vi "LDRLouise.vi"() -> ()   [LabVIEW 2015]
uses:
  <vilib>/Math Plots/2D Math Plots/2D Compass/2D Compass XCtrl/2D Compass.xctl
  <vilib>/Math Plots/2D Math Plots/2D Compass/2D Compass Datatype/Public/Plot Helper (Complex).vi
  <vilib>/Math Plots/2D Math Plots/2D Compass/2D Compass Datatype/2D Compass Datatype.lvclass
panel:
  out "2D Compass":refnum<class "2D Plot Datatype.lvclass">[](xcontrol)
  in  "Channel X":tag="Dev1/ai0"
  in  "Channel Y":tag="Dev1/ai1"
  out "error out":errorcluster
  in  "stop":bool
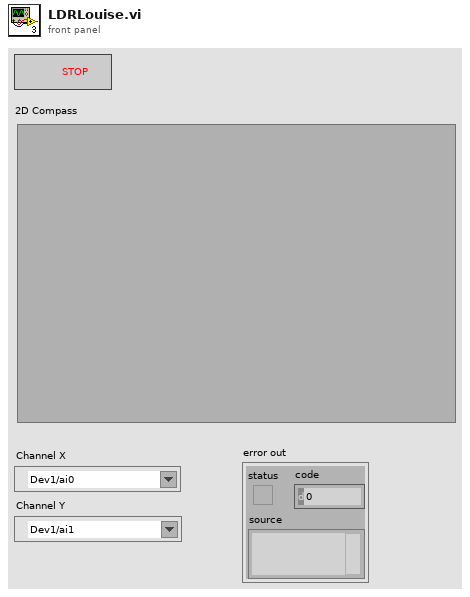
[diagram p1: front panel]
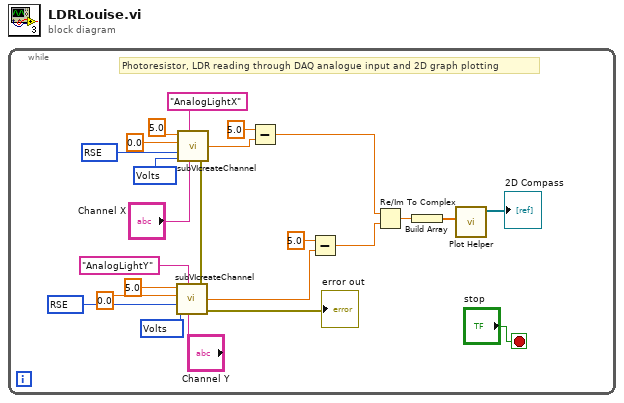
[diagram p0: block diagram]
diagram:
  n1 = while {
    stop <- "stop" stop-if-true
    w3 = 10083 items=["Default"=-1, "RSE"=10083, "NRSE"=10078, "Differential"=10106, "Pseudodifferential"=12529] ("input terminal configuration")
    w4 = 10348 items=["Volts"=10348, "From Custom Scale"=10065] ("units")
    w15 = 10083 items=["Default"=-1, "RSE"=10083, "NRSE"=10078, "Differential"=10106, "Pseudodifferential"=12529] ("input terminal configuration")
    w14 = 10348 items=["Volts"=10348, "From Custom Scale"=10065] ("units")
    # "Photoresistor, LDR reading through DAQ analogue input and 2D graph plotting"
    n2 = call "subVIcreateChannel.vi"("maximum value"=5.0, "name to assign"="AnalogLightX" ("Name X"), "minimum value"=0.0, "input terminal configuration"=w15, "physical channels"="Channel X", "units"=w14) -> ("data"=w16:dbl, "error out"=w13:errorcluster)  [unwired: 1 in]
    n3 = call "subVIcreateChannel.vi"("maximum value"=5.0, "name to assign"="AnalogLightY" ("Name Y"), "minimum value"=0.0, "input terminal configuration"=w3, "physical channels"="Channel Y", "units"=w4, "error in"=w13) -> ("data"=w10:dbl, "error out"=→"error out":errorcluster)
    n4 = Subtract(x=5.0, y=w16) -> (x-y=w1:dbl)
    n5 = Subtract(x=5.0, y=w10) -> (x-y=w2:dbl)
    n6 = Re/Im To Complex(1:w2, 2:w1) -> (0:w23:cdb)
    n7 = Build Array(w23) -> (w22:cdb[])
    n8 = call-poly <vilib>:"Plot Helper.vi"("z vector"=w22) -> ("2D Plot Class Obj Array out"=→"2D Compass":refnum<class "2D Plot Datatype.lvclass">[])  [unwired: 2 in, 8 out]
  }
